vi "converter_V2.0.vi"() -> ()   [LabVIEW 2014]
uses:
  <vilib>/Utility/xml.llb/Read From XML File(string).vi
panel:
  out "Datenspeicher 2":T1={"Fahrzeugdaten"="", "date/time string"="", "Rolle [Inkr/U]"=0, "Rollenumfang [m]"=0.0, "Rollenträgheit [kgm²]"=0.0, "Zündung [Imp/U]"=0, "Getriebe [1:]"=0.0, "Reifenumfang [m] "=0.0, "element"=0.0, "Gl. Mittelwert"=0, "Differenzenquotient"=0, "Polynom"=0, "element"=0.0, "element"=0.0, "Lufttemperatur [°C]"=0.0, "Luftfeuchtigkeit [%]"=0.0, "Luftdruck [mbar]"=0.0, [], [], "Best Polynomial Fit"=[], [], "Übersetzung ermitteln aus"=0, "[s]"=0.0, "nmin [1/min]"=0.0, "nmax [1/min]"=0.0, "n vom Gas [1/min]"=0.0, [], [], "Boolesch"=FALSE, "Serielle Schnittstelle"="COM4"}
  out "Datenspeicher":T2={"Fahrzeugdaten"="", "date/time string"="", "Rolle [Inkr/U]"=0, "Rollenumfang [m]"=0.0, "Rollenträgheit [kgm²]"=0.0, "Zündung [Imp/U]"=0.0, "Getriebe [1:]"=0.0, "Reifenumfang [m] "=0.0, "element"=0.0, "Gl. Mittelwert"=0, "Differenzenquotient"=0, "Polynom"=0, "element"=0.0, "element"=0.0, "Lufttemperatur [°C]"=0.0, "Luftfeuchtigkeit [%]"=0.0, "Luftdruck [mbar]"=0.0, [], [], "Best Polynomial Fit"=[], [], "Übersetzung ermitteln aus"=0, "[s]"=0.0, "nmin [1/min]"=0.0, "nmax [1/min]"=0.0, "n vom Gas [1/min]"=0.0, [], [], "Boolesch"=FALSE, "Serielle Schnittstelle"="COM4", "nKuWe/nRolle"=10.0}
  # "WildBugChilGru XML Converter"
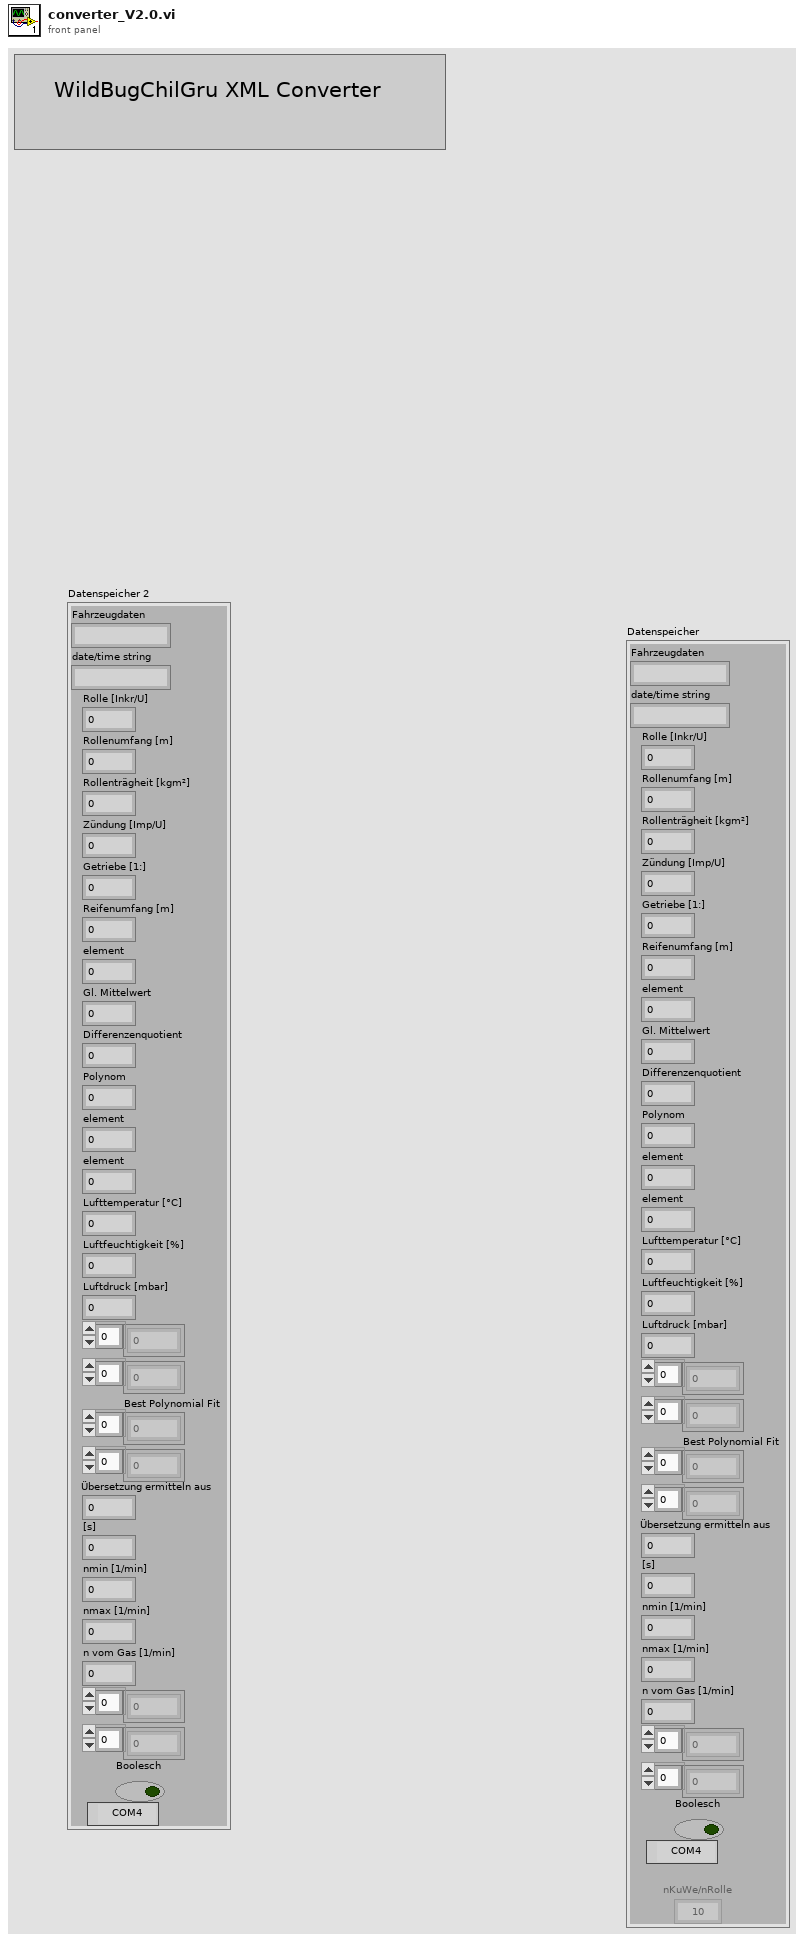
[diagram p1: front panel]
types:
  T1 = cluster{"Fahrzeugdaten":string, "date/time string":string, "Rolle [Inkr/U]":u16, "Rollenumfang [m]":dbl, "Rollenträgheit [kgm²]":dbl, "Zündung [Imp/U]":u8, "Getriebe [1:]":dbl, "Reifenumfang [m] ":dbl, "element":dbl, "Gl. Mittelwert":u8, "Differenzenquotient":u8, "Polynom":u8, "element":dbl, "element":dbl, "Lufttemperatur [°C]":dbl, "Luftfeuchtigkeit [%]":dbl, "Luftdruck [mbar]":dbl, dbl[], dbl[], "Best Polynomial Fit":dbl[], dbl[], "Übersetzung ermitteln aus":u8, "[s]":dbl, "nmin [1/min]":dbl, "nmax [1/min]":dbl, "n vom Gas [1/min]":dbl, dbl[], i32[], "Boolesch":bool, "Serielle Schnittstelle":refnum<visa-resource-name>}
  T2 = cluster{"Fahrzeugdaten":string, "date/time string":string, "Rolle [Inkr/U]":u16, "Rollenumfang [m]":dbl, "Rollenträgheit [kgm²]":dbl, "Zündung [Imp/U]":dbl, "Getriebe [1:]":dbl, "Reifenumfang [m] ":dbl, "element":dbl, "Gl. Mittelwert":u8, "Differenzenquotient":u8, "Polynom":u8, "element":dbl, "element":dbl, "Lufttemperatur [°C]":dbl, "Luftfeuchtigkeit [%]":dbl, "Luftdruck [mbar]":dbl, dbl[], dbl[], "Best Polynomial Fit":dbl[], dbl[], "Übersetzung ermitteln aus":u8, "[s]":dbl, "nmin [1/min]":dbl, "nmax [1/min]":dbl, "n vom Gas [1/min]":dbl, dbl[], i32[], "Boolesch":bool, "Serielle Schnittstelle":refnum<visa-resource-name>, "nKuWe/nRolle":dbl}
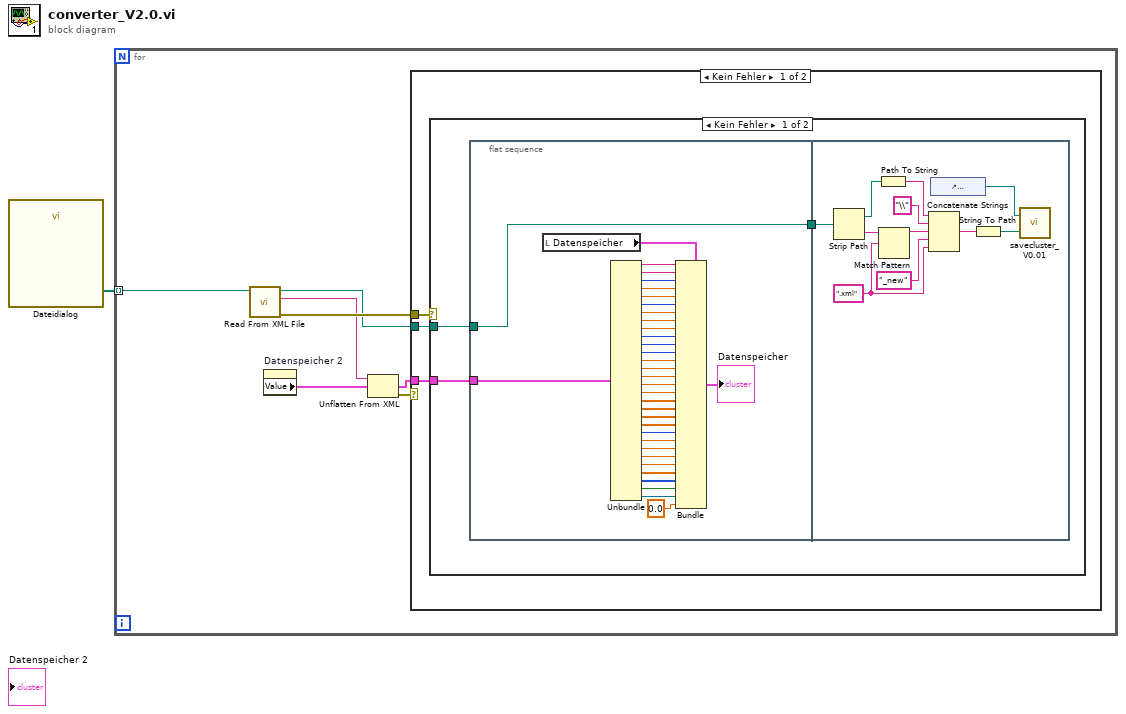
[diagram p0: block diagram]
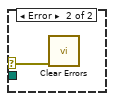
[diagram p2: hidden frame]
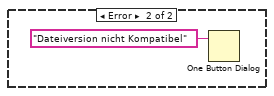
[diagram p3: hidden frame]
diagram:
  n1 = call "Dateidialog"() -> ("selected paths"=w1:path[])  [unwired: 12 in, 3 out]
  n2 = for {
    tunnel: w1 -> [w6] mode=indexing
    n3 = call-poly <vilib>:"Read From XML File.vi"("XML File Path"=w6) -> ("error out"=w8:errorcluster, "XML Elements"=w5:string, "XML File Path(duplicate)"=w7:path)  [unwired: 8 in]
    n4 = property on="Datenspeicher 2" class="Cluster (strikt)"() -> ("Value"=w4:T1)  [unwired: 2 in, 2 out]
    n5 = Unflatten From XML(xml string=w5, type=w4) -> (value=w3:T1, error out=w2:errorcluster)  [unwired: 1 in]
    n6 = case shown="Kein Fehler" w2 {
      tunnel: w8 -> [w11 _]
      tunnel: w7 -> [w10 _]
      tunnel: w3 -> [w9 _]
      frame No Error {
        n7 = case shown="Kein Fehler" w11 {
          selector: w11 -> [_ w61]
          tunnel: w10 -> [w13 _]
          tunnel: w9 -> [w12 _]
          frame No Error {
            n8 = flat-sequence {
              tunnel: w12 -> [w15]
              tunnel: [w16] -> w14
              tunnel: w13 -> [w16]
              tunnel: w14 -> [w60]
              frame #0 {
                n9 = local read "Datenspeicher"() -> (w48:T2)
                n10 = Unbundle(w15) -> ("Fahrzeugdaten"=w47:string, "date/time string"=w46:string, "Rolle [Inkr/U]"=w45:u16, "Rollenumfang [m]"=w44:dbl, "Rollenträgheit [kgm²]"=w18:dbl, "Zündung [Imp/U]"=w19:u8, "Getriebe [1:]"=w20:dbl, "Reifenumfang [m]"=w21:dbl, "element"=w22:dbl, "Gl. Mittelwert"=w23:u8, "Differenzenquotient"=w24:u8, "Polynom"=w25:u8, "element"=w26:dbl, "element"=w27:dbl, "Lufttemperatur [°C]"=w28:dbl, "Luftfeuchtigkeit [%]"=w29:dbl, "Luftdruck [mbar]"=w30:dbl, w31:dbl[], w32:dbl[], "Best Polynomial Fit"=w33:dbl[], w34:dbl[], "Übersetzung ermitteln aus"=w35:u8, "[s]"=w36:dbl, "nmin [1/min]"=w37:dbl, "nmax [1/min]"=w38:dbl, "n vom Gas [1/min]"=w39:dbl, w40:dbl[], w41:i32[], "Boolesch"=w42:bool, "Serielle Schnittstelle"=w43:refnum<visa-resource-name>)
                n11 = Bundle(cluster=w48, "Fahrzeugdaten"=w47, "date/time string"=w46, "Rolle [Inkr/U]"=w45, "Rollenumfang [m]"=w44, "Rollenträgheit [kgm²]"=w18, "Zündung [Imp/U]"=w19, "Getriebe [1:]"=w20, "Reifenumfang [m]"=w21, "element"=w22, "Gl. Mittelwert"=w23, "Differenzenquotient"=w24, "Polynom"=w25, "element"=w26, "element"=w27, "Lufttemperatur [°C]"=w28, "Luftfeuchtigkeit [%]"=w29, "Luftdruck [mbar]"=w30, w31, w32, "Best Polynomial Fit"=w33, w34, "Übersetzung ermitteln aus"=w35, "[s]"=w36, "nmin [1/min]"=w37, "nmax [1/min]"=w38, "n vom Gas [1/min]"=w39, w40, w41, "Boolesch"=w42, "Serielle Schnittstelle"=w43, "nKuWe/nRolle"=0.0) -> (→"Datenspeicher":T2)
              }
              frame #1 {
                w54 = ".xml" ("Regulärer Ausdruck")
                n12 = Strip Path(path=w60) -> (stripped path=w56:path, name=w59:string)
                n13 = Path To String(path=w56) -> (string=w52:string)
                n14 = Match Pattern(string=w59, regular expression=w54) -> (before substring=w51:string)  [unwired: 1 in, 3 out]
                n15 = Concatenate Strings(w52, "\\", w51, "_new" ("String"), w54) -> (w57:string)
                n16 = control-ref of="Datenspeicher"() -> (w53:refnum<vi>)
                n17 = String To Path(string=w57) -> (path=w55:path)
                n18 = call "savecluster_V0.01.vi"("selected path"=w55, "Datenspeicher 3"=w53) -> ()  [unwired: 1 in]
              }
            }
          }
          frame Error {
            n19 = call <vilib>:"Clear Errors.vi"("error in (no error)"=w61) -> ()  [unwired: 5 in, 2 out]
          }
        }
      }
      frame Error {
        n20 = One Button Dialog(message="Dateiversion nicht Kompatibel" ("Nachricht")) -> ()  [unwired: 1 in, 1 out]
      }
    }
  }
